vi "HFRR ADV v01.vi"() -> ()   [LabVIEW 2023] (continued)
5.386904015272106, 5.52926545136433, 5.687444824800141, 5.8368364552672976, 5.9967733772968375, 6.30610192979353, 6.478341691979186, 6.643551259789921, 6.808760827600658, 6.965182652442734, 7.137422414628394, 7.29032914228301, 7.492447230562097, 7.636566215248059, 7.747291776653125, 7.900198504307739, 8.067165620712203, 8.197224216648312, 8.429220631020835, 8.585642455862914, 8.749094475079918, 8.949455014765274, 9.075998513513923, 9.239450532730922, 9.40817519772912, 9.559324376790004, 9.675322583976262, 9.866895380692966, 9.9758633935043, 10.13580031553384, 10.293979688969653, 10.429310930686956, 10.59276294990396, 10.649004504903356, 10.823001815682744, 10.90209150240065, 11.049725584274075, 11.228995540834658, 11.366084331145693, 11.508445767237916, 11.642019460361494, 11.768562959110136, 11.905651749421176, 12.065588671450715, 12.241343530823832, 12.371402126759948, 12.585823055195151, 12.606913638319927, 12.867030830192144, 13.185147125657501, 13.396052956905242, 13.603443690965518, 13.83192500815058, 14.789788991734092, 17.011330414210352, 16.030618298908333, 15.981406938283856, 16.07455701375161, 15.802136981723274, 15.800379433129542, 16.00425507000236, 16.248554324531, 16.299523233749206, 16.77757645124409, 17.11151068405303, 16.812727423118723, 17.187085273583474, 16.94630111624229, 17.89713490545088, 18.072889764823994, 17.842650899045214, 17.6563507481097, 17.695016817171783, 17.872529225138642, 17.911195294200724, 17.890104711075956, 18.043011438730566, 17.958649106231476, 18.048284084511764, 18.072889764823994, 18.004345369668485, 18.148464354354438, 18.1801002290416, 18.17131248607295, 18.25040217279085, 18.257432367165777, 18.31367392216517, 18.35058244263353, 18.403308900445467, 18.41561174060159, 18.392763608883076, 18.459550455444862, 18.4841561357571, 18.507004267475608, 18.51930710763173, 18.57203356544366, 18.58960905138097, 18.619487377474403, 18.642335509192907, 18.64936570356783, 18.60718453731829, 18.605426988724552, 18.59839679434963, 18.57730621122485, 18.59488169716217, 18.56500337106873, 18.55797317669381, 18.57027601684993, 18.56676091966247, 18.531609947787846, 18.538640142162766, 18.528094850600382, 18.521064656225455, 18.52985239919411, 18.5122769132568, 18.482398587163367, 18.605426988724552, 18.614214731693213, 18.56148827388127, 18.56500337106873, 18.57203356544366, 18.549185433725157, 18.540397690756503, 18.52985239919411, 18.52985239919411, 18.5122769132568, 18.51403446185053, 18.515792010444265, 18.482398587163367, 18.494701427319487, 18.475368392788447, 18.464823101226052, 18.443732518101285, 18.459550455444862, 18.44900516388247, 18.427914580757704, 18.45076271247621, 18.436702323726358, 18.42439948357024, 18.433187226538898, 18.427914580757704, 18.408581546226657, 18.41385419200785, 18.389248511695616, 18.398036254664273, 18.38573341450815, 18.38221831732069, 18.38221831732069, 18.35058244263353, 18.368157928570838, 18.348824894039797, 18.34706734544607, 18.340037151071144, 18.331249408102487, 18.327734310915027, 18.31543147075891, 18.31543147075891, 18.301371082009055, 18.287310693259204, 18.297855984821588, 18.280280498884274, 18.275007853103087, 18.269735207321887, 18.25567481857205, 18.252159721384576, 18.232826686853535, 18.239856881228466, 18.215251200916224, 18.217008749509954, 18.209978555135034, 18.19064552060399, 18.195918166385184, 18.183615326229067, 18.169554937479216, 18.17307003466668, 18.153737000135635, 18.151979451541898, 18.137919062792054, 18.125616222635934, 18.12737377122967, 18.115070931073546, 18.115070931073546, 18.10276809091743, 18.099252993729966, 18.095737896542506, 18.09046525076131, 18.081677507792655, 18.067617119042804, 18.062344473261614, 18.055314278886687, 18.044768987324296, 18.03598124435564, 18.032466147168176, 18.023678404199522, 18.025435952793252, 18.021920855605796, 18.00961801544967, 17.99907272388729, 17.997315175293558, 17.99204252951236, 17.98501233513744, 17.97095194638759, 17.963921752012663, 17.958649106231476, 17.953376460450276, 17.946346266075352, 17.934043425919235, 17.93580097451296, 17.97095194638759, 17.953376460450276, 17.955134009044006, 17.94283116888789, 17.93931607170043, 17.927013231544308, 17.921740585763114, 17.891862259669683, 17.895377356857146, 17.89889245404461, 17.893619808263416, 17.881316968107296, 17.88307451670103, 17.879559419513566, 17.865499030763715, 17.833863156076553, 17.837378253264013, 17.80925747576432, 17.796954635608202, 17.796954635608202, 17.78465179545208, 17.77234895529596, 17.767076309514763, 17.777621601077154, 17.774106503889694, 17.742470629202533, 17.768833858108493, 17.719622497484025, 17.724895143265222, 17.724895143265222, 17.7178649488903, 17.728410240452682, 17.707319657327908, 17.70028946295298, 17.716107400296565, 17.703804560140444, 17.677441331234476, 17.65107810232851, 17.66865358826582, 17.5772610613918, 17.53859499232971, 17.52277705498613, 17.52453460357986, 17.515746860611202, 17.51047421483001, 17.50871666623628, 17.49992892326762, 17.491141180298964, 17.480595888736577, 17.477080791549124, 17.466535499986733, 17.464777951393007, 17.45423265983061, 17.44720246545569, 17.43314207670584, 17.43489962529957, 17.43138452811211, 17.419081687955984, 17.4085363963936, 17.403263750612407, 17.403263750612407, 17.390960910456286, 17.38744581326883, 17.382173167487633, 17.368112778737785, 17.368112778737785, 17.35405238998793, 17.347022195613008, 17.34174954983182, 17.339992001238087, 17.329446709675697, 17.325931612488237, 17.31714386951958, 17.308356126550922, 17.304841029363462, 17.303083480769722, 17.29429573780107, 17.278477800457495, 17.2732051546763, 17.26969005748884, 17.26265986311391, 17.257387217332717, 17.252114571551527, 17.245084377176603, 17.239811731395402, 17.23805418280167, 17.223993794051825, 17.223993794051825, 17.22047869686436, 17.213448502489445, 17.209933405301975, 17.20290321092705, 17.192357919364667, 17.188842822177204, 17.178297530614817, 17.17478243342735, 17.15720694749004, 17.146661655927648, 17.14490410733392, 17.136116364365265, 17.12908616999034, 17.122055975615414, 17.113268232646764, 17.178297530614817, 17.162479593271232, 17.115025781240494, 17.08338990655333, 17.081632357959595, 17.081632357959595, 17.067571969209745, 17.067571969209745, 17.06054177483482, 17.05702667764736, 17.051754031866164, 17.042966288897507, 17.035936094522594, 17.02363325436647, 17.01484551139781, 17.00957286561662, 16.995512476866768, 16.991997379679308, 16.990239831085574, 16.98496718530438, 16.979694539523184, 16.977936990929454, 16.96387660217961, 16.95508885921095, 16.951573762023486, 16.94278601905482, 16.933998276086164, 16.933998276086164, 16.92169543593005, 16.91642279014886, 16.9129076929614, 16.91642279014886, 16.904119949992744, 16.897089755617817, 16.895332207024087, 16.88654446405543, 16.87775672108677, 16.883029366867966, 16.867211429524385, 16.858423686555728, 16.85490858936826, 16.846120846399604, 16.832060457649764, 16.83030290905603, 16.823272714681107, 16.81624252030618, 16.810969874524982, 16.802182131556325, 16.8004245829626, 16.789879291400208, 16.789879291400208, 16.781091548431554, 16.768788708275437, 16.770546256869167, 16.767031159681704, 16.756485868119317, 16.754728319525583, 16.745940576556933, 16.738910382182006, 16.733637736400812, 16.724849993432162, 16.716062250463505, 16.702001861713647, 16.69672921593246, 16.698486764526187, 16.684426375776336, 16.682668827182606, 16.677396181401413, 16.666850889839022, 16.661578244057836, 16.659820695464106, 16.64927540390171, 16.640487660933058, 16.633457466558134, 16.628184820776944, 16.622912174995744, 16.622912174995744, 16.615881980620824, 16.60533668905843, 16.600064043277243, 16.59830649468351, 16.5807310087462, 16.577215911558728, 16.573700814371275]
  in  "ENTER THE NEW PASSWORD":string caption="Enter The New Password"
  in  "ENTER CURRENT PASSWORD":string caption="Enter Current Password"
  out "Port 3 Error":errorcluster
  in  "Lubrication System COM Port :":refnum<visa-resource-name>="COM9" caption="Ambient Temperature COM Port:"
  in  "LvdtOff":dbl=2.875 caption="LVDT Position Offset :" min=2.1 max=2.9 format="%.4f"
  out "Port 2 Error":errorcluster={"status"=TRUE, "code"=-1073807343, "source"="Property Node (arg 1) in VISA Configure Serial Port (Instr).vi->Winducom 2010--std ed hfrr-wo1768-V18.vi"}
  out "Port 1 Error":errorcluster={"status"=TRUE, "code"=-1073807343, "source"="Property Node (arg 1) in VISA Configure Serial Port (Instr).vi->Winducom 2010--std ed hfrr-wo1768-V18.vi"}
  in  "Stroke PID Gains":T9={"Proportional Gain (Kc)"=200.0, "Integral Time (Ti, min)"=0.02, "Derivative Time (Td, min)"=0.0}
  in  "CH-HUMIDITY DRY":u16=3 caption="Ch-Humidity Wet:" max=7 step=1
  in  "CH-HUMIDITY WET":u16=4 caption="Ch-Humidity Dry:" max=7 step=1
  in  "CH-HEATER":u16=2 caption="Ch-Heater:" max=7 step=1
  in  "CH-POWER -":u16=1 caption="Ch-Power -:" max=7 step=1
  in  "CH-POWER +":u16 caption="Ch-Power +:" max=7 step=1
  out "String 4":string
  in  "Com Port 3":refnum<visa-resource-name>="COM4" caption="Port 3"
  in  "Prog Due":bool
  in  "Prog Uno":bool
  in  "Com Port 2":refnum<visa-resource-name>="COM7" caption="Port 2:"
  in  "Com Port 1":refnum<visa-resource-name>="COM5" caption="Port 1:"
  in  "message":string="*Entered password is wrong"
  in  "SPEED OUT:":dbl=1.0 caption="Speed Out:" min=0.0001 max=5.0 step=0.0001 format="%.4f"
  in  "Temperature before test 3":dbl caption="Temp Before Test" format="%#_5g"
  in  "Humidity before test 3":dbl caption="Humidity Before Test" format="%#_5g"
  out "Temperature after test 5":dbl caption="Temp Before Test" format="%#_5g"
  out "Temperature after test 4":dbl caption="Temp After Test" format="%#_5g"
  out "Humidity after test 4":dbl caption="Humidity After Test ( % Rh )" format="%#_5g"
  out "Humidity before test 4":dbl caption="Humidity Before Test ( % Rh )" format="%#_5g"
  in  "Tab Control 9":enum32{"Page 1", "Page 2"}(tab)
  out "Ref B Scar Value :":string caption="Reference Fluid Information"
  out "Ref B Test Date :":string caption="Reference Fluid Information"
  out "Ref A Scar Value :":string caption="Reference Fluid Information"
  out "Ref A Test Date :":string caption="Reference Fluid Information"
  out "XY Graph 16":cluster{dbl[], dbl[]}[](graph)
  out "TITTLE 4":string caption="Reference Fluid Information"
  out "Sample ID  7":string caption="Fuel Name :"
  out "Sample ID  6":string caption="Fuel Type :"
  out "Mean Wear ( microns) :":dbl format="%#.6f"
  out "Wear Scar Y ( microns ) :":dbl format="%#.6f"
  out "Length ( microns ) 2":dbl caption="Wear Scar X ( microns ) :" format="%#.6f"
  out "s.NO 2":string caption="Instrument  S.NO :"
  out "Test Date 2":string caption="Tested date :"
  out "Tested by 2":string caption="Tested by :"
  out "Sample ID  2":string caption="Sample ID :"
  out "TITTLE 2":string caption="File Name :"
  in  "EDIT 3":bool
  in  "Upload Rate (s)":dbl=1.0 min=0.5 max=5.0 step=0.5 format="%.1g"
  in  "Secret Key":string="22gKHnAGFaJhuNtaR9srYhcD6RQR8M7Zp2xk4ssPTuwGqWUBv7WxW7cXAFkFFbns"
  in  "Serial No":string="HFRR2391"
  in  "Model No":string="MD987654325"
  in  "Data File Name":string="JSON_Single_Point.JSON"
  in  "Path":path=path "C:/LAB-IQ-NXT"
  in  "Upld AR 2":bool
  in  "Sen.Upload Rate (s)":dbl=5.0 min=0.5 max=5.0 step=0.5 format="%.1g"
  in  "Run test 3":bool
  in  "Sensor File Name":string="JSON_Health.JSON"
  in  "Upld AR":bool
  in  "Total No. of Tests":dbl
  in  "Tab Control 6":enum32{"Data", "Sensor"}(tab)=enum."Sensor"
  out "Respose From Server":string
  out "standard output":string
  out "SinglePoint":string
  in  "JSON Check String":string="\"Stored\": true"
  in  "JSONH Check String":string="\"Stored\": true"
  out "standard output 2":string
  in  "Sensor Information":string[][](array[string])=[["Sensor Name", "Sensor Model Number", "Sensor Run time Hours", "Sensor State"], ["Normal Load Sensor", "MPF-AC20-X3U791", "", ""], ["Frictional Force Sensor", "MPF-AC20-X3U792", "", ""], ["Temperature Sensor", "MPF-AC20-X3U793", "", ""], ["Speed Sensor", "MPF-AC20-X3U794", "", ""], ["LVDT Sensor", "MPF-AC20-X3U795", "", ""], ["Vibration Sensor ", "MPF-AC20-X3U796", "", ""]]
  out "Respose From Server 2":string
  out "FF buffer":dbl[](graph)
  out "%  o/p":dbl
  out "sample4":dbl format="%_4f"
  out "freq 4":dbl format="%_4f"
  out "conststatus":dbl=10.0 min=0.0 max=200.0 step=1.0
  out "CP4":dbl=nan min=0.0 max=200.0 step=0.1 format="%.3f"
  out "CP3":dbl=nan min=0.0 max=200.0 step=0.1 format="%.3f"
  out "Boolean  4":bool=TRUE caption="Power Status"
  in  "Boolean BC T & BG 2":cluster{u32, u32}[](array[cluster])=[{3158064, 16250871}, {11918296, 8965631}]
  in  "GBG   2":u32(colorbox)=16250871 caption="Graph Background"
  in  "GFG  2":u32(colorbox)=8964095 caption="Graph Foreground"
  in  "GBG":u32(colorbox)=16250871 caption="Graph Background"
  in  "GFG":u32(colorbox)=8964095 caption="Graph Foreground"
  in  "Boolean BC T & BG":cluster{u32, u32}[](array[cluster])=[{3158064, 16250871}, {11918296, 8965631}]
  in  "SC  Text":u32(colorbox) caption="String Control Text"
  in  "SC BG 3":u32(colorbox)=16777215 caption="String Control BG"
  in  "NI BG 2":u32(colorbox)=13553358 caption="Numeric Indicator BG"
  in  "NI Text  2":u32(colorbox)=7105644 caption="Numeric Indicator Text"
  in  "NC Text":u32(colorbox)=3381759 caption="Numeric Control Text"
  in  "NC BG":u32(colorbox)=16777215 caption="Numeric Control BG"
  out "ABS DP":dbl[](graph)
  in  "Com flag":u32
  out "Gain path":string="C:\\Winducom 2010\\STD ED HFRR\\wo1768"
  out "String 45":string="S.NO"
  out "String 44":string
  out "error out 4":errorcluster
  out "concatenated string 2":string
  out "String 42":string
  out "error out 3":errorcluster
  out "STR":string
  out "gain":string
  out "export":string
  out "before substring":string
  out "output":string
  out "test by":string
  out "export 2":string
  out "export":string
  out "REMARKS 2":string="@WINDUCOM : RECIPROCATORY TEST RIG    DEFINITON FILE       \r  Sample ID :- , Load :-  2.00 N , Remarks :- , Date :- 05/11/2016, 06:04\r"
  out "data":string
  out "Boolean 3":bool
  out "String 41":string=":-@(WINDUCOM : RECIPROCATORY TEST RIG    DEFINITON FILE )      "
  out "concatenated string":string
  out "path":path
  out "String 40":string
  out "Boolean 2":bool=TRUE
  in  "Set Rh 2":dbl=50.0 caption="HUMIDITY" min=35.0 max=85.0 step=1.0
  out "String 39":string="WS1.4="
  out "String 38":string="HCF="
  out "String 37":string="MWSD="
  out "String 36":string="AVP ="
  out "String 35":string="Temp after test="
  out "String 34":string="Temp before test="
  out "String 33":string="Tested by"
  out "String 32":string="Sample ID "
  out "String 31":string="Tested date"
  out "String 30":string="Sample Design"
  out "path string":string
  out "String 29":string
  out "St. Line eqn : 2":string
  out "Numeric 10":i32
  out "Numeric 16":i32
  out "S 106":string="Off"
  out "S 105":string="On"
  out "S 104":string="Heater Off"
  out "S 103":string="Heater On"
  out "S 102":string="Ch-Humidity Dry:"
  out "S 101":string="Ch-Humidity Wet:"
  out "S 100":string="Ch-Heater:"
  out "S 99":string="Ch-Power -:"
  out "S 98":string="Ch-Power +:"
  out "S 97":string="Port 2"
  out "S 96":string="Port 1"
  out "S 95":string="Stroke Gain :"
  out "S 94":string="Displacement :"
  out "S 93":string="Stop"
  out "S 92":string="Run"
  in  "LAnguage":enum32{"Page 1", "Page 2"}(tab)
  out "S 91":string="Threshold"
  out "S 90":string="File path"
  out "S 89":string="Newtons ( N )"
  out "S 88":string="Change Calibrate Password"
  out "S 87":string="Enter The New Password"
  out "S 86":string="Enter Current Password"
  out "S 85":string="Password"
  out "S 84":string="Save Gain Constants"
  out "S 83":string="Air Temperature ( deg C )"
  out "S 82":string="TIME ( mins )"
  out "S 81":string="Relative Humidity ( Rh )"
  out "S 80":string="Sample TEMPERATURE ( Deg C)"
  out "S 79":string="Stroke"
  out "S 78":string="Air Temperature"
  out "S 77":string="mm"
  out "S 76":string="Stroke"
  out "S 75":string="WINDUCOM 2010 \\XXXX\\VX.XX\\MONTH YEAR"
  out "S 74":string="Frictional Force ( N )"
  out "S 73":string="Calibrate Parameter"
  out "S 72":string="Save Gain Constant"
  out "S 71":string="Edit Gain Constant"
  out "S 70":string="Humidity :"
  out "S 69":string="Air Temperature :"
  out "S 68":string="Speed Out:"
  out "S 67":string="Temperature :"
  out "S 66":string="Frictional Force :"
  out "S 65":string="ABOUT"
  out "S 64":string="Frictional  Force ( N )"
  out "S 63":string="Temperature ( Deg C)"
  out "S 62":string="Time ( mins )"
  out "S 60":string="Reset Graph"
  out "S 59":string="COF4"
  out "S 58":string="COF3"
  out "S 57":string="COF2"
  out "S 56":string="COF1"
  out "S 55":string="Frictional Force ( N )"
  out "S 54":string="Temperature"
  out "S 53":string="Coefficient Of Friction"
  out "S 52":string="Refresh"
  out "S 51":string="File 4"
  out "S 50":string="File 3"
  out "S 49":string="File 2"
  out "S 48":string="File 1"
  out "S 47":string="COMPARE FILES"
  out "S 46":string="SAVE RESULT"
  out "S 45":string="WS1.4"
  out "S 44":string="HCF"
  out "S 43":string="MWSD"
  out "S 42":string="AVP "
  out "S 41":string
  out "S 40":string
  out "S 39":string="Humidity after test="
  out "S 38":string="Humidity before test="
  out "S 37":string
  out "S 36":string="Rh Before"
  out "S 35":string="ISO : WS1.4"
  out "S 34":string="FRICTIONAL FORCE ( N )"
  out "S 33":string="Reset Graph"
  out "S 32":string="Data points"
  out "S 31":string="COEFFICIENT OF FRICTION"
  out "S 30":string="RUN"
  out "S 29":string="Test Status"
  out "S 28":string="Power"
  out "S 27":string="Engage"
  out "S 26":string="Present ( Sec )"
  out "S 25":string="Count down ( sec )"
  out "S 24":string="Sec"
  out "S 23":string="Save Dwell"
  out "S 22":string="Elapsed Time"
  out "S 21":string="min"
  out "S 20":string="Test duration"
  out "S 19":string="TIMER"
  out "S 18":string="OFF"
  out "S 17":string="Rh"
  out "S 16":string="HUMIDITY"
  out "S 15":string="Heater On"
  out "S 14":string="TEMPERATURE ( Deg C)"
  out "S 13":string="N"
  out "S 12":string="NORMAL LOAD"
  out "S 11":string="Hz"
  out "S 10":string="FREQUENCY"
  out "S 9":string="STOP"
  out "S 8":string="STAND BY"
  out "S 7":string="Remarks :"
  out "S 6":string="Sample ID :"
  out "S 5":string="File Name :"
  out "S 4":string="Acquire"
  out "S 3":string="EXIT"
  out "S 2":string="Winducom 2010"
  out "S":string="ENGLISH TITLES"
  out "Error Due":errorcluster={"status"=TRUE, "code"=-1073807343, "source"="Property Node (arg 1) in VISA Configure Serial Port (Instr).vi->Winducom 2010--std ed hfrr-wo1768-V18.vi"}
  out "Error Uno":errorcluster={"status"=TRUE, "code"=-1073807343, "source"="Property Node (arg 1) in VISA Configure Serial Port (Instr).vi->Winducom 2010--std ed hfrr-wo1768-V18.vi"}
  out "as":string
  out "bs":string="Rh After"
  out "as":string=" after test"
  out "bs":string="Temp"
  out "as":string=" before test"
  out "bs":string="Temp"
  out "as":string=" after test"
  out "bs":string
  out "bs":string="Humidity"
  out "as":string=" before test"
  out "bs":string="Humidity"
  out "S 61":string="Frictional Force ( N )"
  in  "Lan flag":dbl=22.0
  in  "Table":string[][](table)=[["ENGLISH TITLES", "RUSSIAN"], ["Winducom 2010", "Winducom  2010"], ["Exit", "Выход"], ["Acquire", "ИСПЫТАНИЕ     "], ["File Name :", "Имя файла :"], ["Sample ID :", "Имя образца :"], ["Remarks :", "Примечания :"], ["Standby", "ОЖИДАНИЕ"], ["Stop", "СТОП"], ["Frequency", "ЧАСТОТА"], ["Hz", "Гц"], ["Normal Load", "НАГРУЗКА"], ["N", "Н"], ["Temperature ( Deg C)", "ТЕМПЕРАТУРА (Град С)"], ["Heater On", "НАГРЕВ ВКЛ"], ["Humidity", "ВЛАЖНОСТЬ"], ["Rh", "%"], ["OFF", "ВЫКЛ"], ["Timer", "ВРЕМЯ"], ["Test duration", "ВРЕМЯ ТЕСТА"], ["min", "мин"], ["Elapsed Time", "依商判"], ["Save Dwell", "ИНТЕРВАЛ"], ["Sec", "Сек"], ["Count down ( Sec )", "До запуска (сек)"], ["Present ( Sec )", "Таймер (сек)"], ["Run", "Применить"], ["Power", "ПИТАНИЕ"], ["Test Status", "СТАТУС"], ["Manual Over Ride", "ПУСК"], ["Coefficient Of Friction", "КОЭФФИЦИЕНТ ТРЕНИЯ"], ["Data points", "Точки"], ["Reset Graph", "Сбросить график"], ["Frictional Force ( N )", "СИЛА ТРЕНИЯ (Н)"], ["ISO : WS1.4", "ISO : WS1.4"], ["Rh Before", "Влажность до"], ["Rh After", "Влажность, после"], ["Humidity, before test", "Влажность, до теста"], ["Humidity, after test", "Влажность, после теста"], ["Temp, before test", "Температура, до теста"], ["Temp, after test", "Температура, после теста"], ["AVP ", "СДП"], ["MWSD", "MWSD"], ["HCF", "ФКВ"], ["WS1.4", "WS1.4"], ["Save Result", "Сохранить результат"], ["COMPARE FILES", ""], ["File 1", "ФАЙЛ 1"], ["File 2", "ФАЙЛ 2"], ["File 3", "ФАЙЛ 3"], ["File 4", "ФАЙЛ 4"], ["Refresh", "ОБНОВИТЬ"], ["Coefficient Of Friction", "КОЭФФИЦИЕНТ ТРЕНИЯ"], ["Temperature", "ТЕМПЕРАТУРА"], ["Frictional Force ( N )", "СИЛА ТРЕНИЯ (Н)"], ["COF1", "КОФ1"], ["COF2", "КОФ2"], ["COF3", "КОФ3"], ["COF4", "КОФ4"], ["Reset Graph", "Сбросить график"], ["Time ( mins )", "Время (мин)"], ["Temperature ( Deg C)", "ТЕМПЕРАТУРА (Град С)"], ["Frictional  Force ( N )", "СИЛА ТРЕНИЯ (Н)"], ["ABOUT", ""], ["Frictional Force :", "КОЭФ.ТРЕНИЯ:"], ["Temperature :", "ТЕМПЕРАТУРА"], ["Speed Out:", "СКОРОСТЬ"], ["Air Temperature :", "ТЕМПЕРАТУРА ВОЗДУХА"], ["Humidity :", "ВЛАЖНОСТЬ"], ["Edit Gain Constant", "КОРРЕКТИРОВКА КОНСТАНТ"], ["Save Gain Constant", "СОХРАНИТЬ КОНСТАНТЫ"], ["Calibrate Parameter", "ПАРАМЕТРЫ КАЛИБРОВКИ"], ["Frictional Force ( N )", "СИЛА ТРЕНИЯ (Н)"], ["WINDUCOM 2010 \\XXXX\\VX.XX\\MONTH YEAR", "WINDUCOM 2010 \\XXXX\\VX.XX\\MONTH YEAR"], ["Stroke", "ДЛИННА ХОДА"], ["mm", "мм"], ["Air Temperature", "ВОЗДУХА ТЕМП"], ["Stroke", "ДЛИННА ХОДА "], ["Time ( mins )", "ВРЕМЯ ( мин )"], ["Sample Temperature( Deg C)", "Образец ТЕМПЕРАТУРА (Град С)"], ["Relative Humidity ( Rh )", "Относительный Влажность ( % )"], ["Air Temperature ( deg C )", "ТЕМПЕРАТУРА ВОЗДУХА (Град С)"], ["Save Gain Constants", "СОХРАНИТЬ КОНСТАНТЫ"], ["Password", "ПАРОЛЬ ДОСТУПА"], ["Enter Current Password", "ВВЕДИТЕ ТЕКУЩИЙ ПАРОЛЬ"], ["Enter The New Password", "ВВЕДИТЕ НОВЫЙ ПАРОЛЬ"], ["Change Calibrate Password", "Сбросить пароль калибровки"], ["Newtons ( N )", "Ньютон ( Н )"], ["File path", "Путь к файлу"], ["Threshold", "порог"], ["Run", "ПУСК"], ["Stop", "СТОП"], ["Displacement :", "смещение:"], ["Stroke Gain :", "ДЛИННА ХОДА:"], ["Port 1", "порт 1"], ["Port 2", "порт 2"], ["Ch-Power +:", "CH-ПИТАНИЕ +:"], ["Ch-Power -:", "CH-ПИТАНИЕ -:"], ["Ch-Heater:", "НАГРЕВ:"], ["Ch-Humidity Wet:", "CH-Увлажнение:"], ["Ch-Humidity Dry:", "CH-Осушение:"], ["Heater On", "НАГРЕВ ВКЛ"], ["Heater Off", "НАГРЕВ ВЫКЛ"], ["On", "ВКЛ"], ["Off", "ВЫКЛ"], ["TEXT REPORT", "ПРОТОКОЛ ИСПЫТАНИЯ"], ["Open Data File", "ОТКРЫТЬ ФАЙЛ ДАННЫХ"], ["Refresh", "ОБНОВЛЕНО"], ["Tittle", "заглавие"], ["Sample Design", "Образец"], ["Tested date", "Дата"], ["Sample ID ", "Имя образца"], ["Tested by", "Испытано"], ["System Configured Printers ", "Сконфигурированные принтеры"], ["Selected Printer", "Выбранный принтер"], ["Select Printer 3", "Выбрать  Печать"], ["Print", "Печать"], [":-@(WINDUCOM : RECIPROCATORY TEST RIG    DEFINITON FILE )      ", "(Анализатор HFRR с возвратно-поступательным механизмом для определения смазывающей способности дизельных топлив )"], ["Tested by:", "Оператор:"], ["          TIME;      COF;       STROKE  (mm);     AIR TEMP ( Deg C);  TEMP ( Deg C);  HUMIDITY ( Rh );", "КОЭФФИЦИЕНТ ТРЕНИЯ;   Инсульт; ТЕМПЕРАТУРА ВОЗДУХА; ВЛАЖНОСТЬ;"], ["Export", "Экспорт"], ["Temperature Intercept :", "ТЕМП перехват:"], ["Air Temperature Intercept:", "ТЕМП  ВОЗДУХА перехват:"], ["Select File Type ", "Выберете формат файла"], ["S.NO", "S.NO"], ["Trip", ""]]
  out "Fric Val":dbl[](array[numeric])
  out "FF cal val":dbl[](array[numeric])=[-0.013084344151737926, -0.01288606647100253, -0.011498122705853597, -0.012092955748060075, -0.011101567344382515, -0.011696400386589284, -0.010705011982911433, -0.010110178940704664, -0.011498122705853597, -0.01090328966364712, -0.009911901259969269, -0.009911901259969269, -0.009515345898498478, -0.008523957494820628, -0.008127402133349837, -0.008127402133349837, -0.009118790537027396, -0.008325679814085232, -0.008325679814085232, -0.008523957494820628, -0.008325679814085232, -0.008127402133349837, -0.008523957494820628, -0.00792912445261415, -0.008325679814085232, -0.008325679814085232, -0.007730846771878755, 0.0015882042226915277, -0.0027739047534900835, -0.0059463476452584485, -0.007136013729671986, -0.006739458368200904, -0.008325679814085232, -0.008523957494820628, -0.007334291410407381, -0.007730846771878755, -0.007334291410407381, -0.007136013729671986, -0.00792912445261415, -0.007334291410407381, -0.006937736048936299, -0.006342903006729822, -0.006342903006729822, -0.006342903006729822, -0.006144625325994427, -0.006144625325994427, -0.0055497922837873664, -0.004954959241580889, -0.005351514603051971, -0.004954959241580889, -0.004954959241580889, -0.004161848518639016, -0.003170460114961457, -0.0023773493920190014, -0.0023773493920190014, -0.0019807940305479194, -0.0019807940305479194, -0.0011876833076060467, -0.0009894056268700685, -0.0009894056268700685, -0.0009894056268700685, -0.0007911279461346732, -0.00019629490392819582, 0.00020026045754288624, 0.0007950934997493636, 0.001389926541955841, 0.0021830372648982965, 0.0033727033493112513, 0.004165814072253707, 0.0037692587107826248, 0.0037692587107826248, 0.004165814072253707, 0.0049589247951955795, 0.005752035518137744, 0.006346868560344221, 0.007338256964022072, 0.007734812325493154, 0.008726200729171005, 0.010510699855790728, 0.00991586681358396, 0.011105532897997497, 0.011502088259468288, 0.012096921301675348, 0.012493476663146139, 0.01289003202461722, 0.01289003202461722, 0.014277975789765862, 0.015269364193443713, 0.016260752597121272, 0.01745041868153452, 0.018243529404476683, 0.019036640127418555, 0.018640084765947473, 0.01982975085036101, 0.020028028531096406, 0.021415972296245048, 0.021415972296245048, 0.0224073606999229, 0.023002193742129376, 0.02379530446507154, 0.024984970549484786, 0.025579803591691264, 0.024984970549484786, 0.02538152591095587, 0.025976358953162346, 0.026571191995369114, 0.027166025037575592, 0.027959135760518047, 0.027959135760518047, 0.02875224648345963, 0.029545357206402084, 0.03033846792934425, 0.03033846792934425, 0.030933300971550726, 0.0313298563330221, 0.03212296705596397, 0.03271780009817045, 0.03291607777890643, 0.03470057690552586, 0.034502299224790464, 0.03529540994773234, 0.03668335371288127, 0.036485076032145874, 0.0380712974780302, 0.03727818675508775, 0.03787301979729481, 0.04659723774965803, 0.0406489073275918, 0.04025235196612072, 0.04005407428538532, 0.04104546268906317, 0.041442018050534254, 0.04699379311112911, 0.05155417976804641, 0.05314040121393045, 0.05333867889466584, 0.05433006729834369, 0.05452834497907909, 0.057700787870848036, 0.055718011063492626, 0.047786903834071276, 0.04461446094230262, 0.043821350219360164, 0.043821350219360164, 0.04362307253862477, 0.04421790558083154, 0.04461446094230262, 0.0452092939845091, 0.0450110163037737, 0.0452092939845091, 0.045804127026715866, 0.04600240470745155, 0.04639896006892234, 0.04719207079186451, 0.047390348472600194, 0.04798518151480696, 0.04858001455701315, 0.04937312527995531, 0.05016623600289748, 0.05135590208731072, 0.05135590208731072, 0.05135590208731072, 0.05135590208731072, 0.05155417976804641, 0.05254556817172426, 0.051752457448781805, 0.05155417976804641, 0.05214901281025318, 0.0519507351295172, 0.051752457448781805, 0.05333867889466584, 0.052347290490988574, 0.05254556817172426, 0.05294212353319505, 0.05393351193687261, 0.05393351193687261, 0.053735234256137215, 0.05393351193687261, 0.0541317896176083, 0.054726622659814775, 0.055321455702021544, 0.05551973338275694, 0.05591628874422802, 0.05710595482864156, 0.057304232509376954, 0.05849389859378991, 0.05829562091305422, 0.057700787870848036, 0.05750251019011235, 0.058097343232318535, 0.057304232509376954, 0.057700787870848036, 0.05789906555158343, 0.058097343232318535, 0.058692176274525595, 0.058692176274525595, 0.05928700931673207, 0.05948528699746776, 0.05948528699746776, 0.06087323076261669, 0.06047667540114561, 0.06047667540114561, 0.06087323076261669, 0.06087323076261669, 0.06126978612408748, 0.06126978612408748, 0.06186461916629425, 0.06245945220850073, 0.06206289684702965, 0.06186461916629425, 0.06186461916629425, 0.062261174527765334, 0.06206289684702965, 0.06206289684702965, 0.0632525629314429, 0.06285600756997181, 0.06364911829291427, 0.0630542852507072, 0.06285600756997181, 0.06245945220850073, 0.06265772988923642, 0.06285600756997181, 0.06364911829291427, 0.06384739597364966, 0.06384739597364966, 0.06384739597364966, 0.06384739597364966, 0.06464050669659183, 0.06503706205806291, 0.0652353397387986, 0.06483878437732722, 0.06543361741953399, 0.0652353397387986, 0.0652353397387986, 0.06503706205806291, 0.06563189510026968, 0.06602845046174047, 0.06682156118468263, 0.0676146719076245, 0.06880433799203804, 0.07851994434807912, 0.08149410955911209, 0.0721750585645418, 0.07138194784159993, 0.07019228175718698, 0.07019228175718698, 0.07078711479939345, 0.07019228175718698, 0.07138194784159993, 0.07197678088380641, 0.07257161392601288, 0.07237333624527749, 0.07237333624527749, 0.07356300232969074, 0.0743561130526329, 0.0743561130526329, 0.07415783537189721, 0.07415783537189721, 0.0743561130526329, 0.0745543907333683, 0.07554577913704615, 0.07415783537189721, 0.0745543907333683, 0.07554577913704615, 0.07574405681778183, 0.07594233449851723, 0.07633888985998831, 0.0767354452214591, 0.0765371675407237, 0.07633888985998831, 0.07693372290219479, 0.0765371675407237, 0.0765371675407237, 0.07614061217925233, 0.07614061217925233, 0.07614061217925233, 0.07614061217925233, 0.0765371675407237, 0.07713200058293018, 0.07693372290219479, 0.07693372290219479, 0.07733027826366587, 0.07713200058293018, 0.0765371675407237, 0.0765371675407237, 0.07614061217925233, 0.0765371675407237, 0.0765371675407237, 0.07574405681778183, 0.07554577913704615, 0.07554577913704615, 0.07475266841410427, 0.07574405681778183, 0.0745543907333683, 0.07376128001042642, 0.07356300232969074, 0.07376128001042642, 0.07336472464895534, 0.07395955769116182, 0.0743561130526329, 0.07475266841410427, 0.07495094609483967, 0.0745543907333683, 0.0743561130526329, 0.07356300232969074, 0.07257161392601288, 0.07257161392601288, 0.07376128001042642, 0.07296816928748397, 0.07276989160674857, 0.07276989160674857, 0.07276989160674857, 0.07237333624527749, 0.07257161392601288, 0.07237333624527749, 0.07197678088380641, 0.07177850320307101, 0.07158022552233533, 0.07158022552233533, 0.07177850320307101, 0.07177850320307101, 0.07237333624527749, 0.07257161392601288, 0.07276989160674857, 0.07356300232969074, 0.07356300232969074, 0.07316644696821965, 0.07376128001042642, 0.07376128001042642, 0.0743561130526329, 0.07495094609483967, 0.07554577913704615, 0.07713200058293018, 0.07752855594440126, 0.07812338898660803, 0.07871822202881451, 0.07812338898660803, 0.07832166666734372, 0.08010616579396344, 0.08684760693897126, 0.08248549796278964, 0.08149410955911209, 0.08149410955911209, 0.08169238723984748, 0.08228722028205396, 0.08724416230044234, 0.09398560344545102, 0.09339077040324396, 0.09497699184912858, 0.09596838025280614, 0.09775287937942587, 0.09834771242163234, 0.10033048922898775, 0.1017184329941364, 0.10290809907854964, 0.10469259820516966, 0.10310637675928533, 0.10310637675928533, 0.10330465444002072, 0.10409776516296318, 0.10766676341620263, 0.10786504109693802, 0.1062788196510537, 0.1104426509465002, 0.10766676341620263, 0.10905470718135127, 0.11064092862723589, 0.10905470718135127, 0.10072704459045913, 0.0991408231445748, 0.09973565618678128, 0.09953737850604588, 0.09993393386751667, 0.10013221154825236, 0.10013221154825236, 0.09973565618678128, 0.10033048922898775, 0.10033048922898775, 0.10132187763266531, 0.10132187763266531, 0.10132187763266531, 0.10132187763266531, 0.10211498835560777, 0.10211498835560777, 0.1037012098014921, 0.10270982139781425, 0.10310637675928533, 0.1037012098014921, 0.10429604284369857, 0.10409776516296318, 0.10389948748222749, 0.10469259820516966, 0.10489087588590505, 0.10528743124737643, 0.10568398660884751, 0.10588226428958261, 0.10568398660884751, 0.106080541970318, 0.10647709733178909, 0.10766676341620263, 0.1062788196510537, 0.10687365269326046, 0.10687365269326046, 0.10707193037399586, 0.10707193037399586, 0.10687365269326046, 0.10687365269326046, 0.10727020805473154, 0.10766676341620263, 0.1082615964584091, 0.10806331877767342, 0.10845987413914479, 0.10865815181988048, 0.10964954022355804, 0.11004609558502883, 0.11064092862723589, 0.11143403935017776, 0.11143403935017776, 0.11143403935017776, 0.11222715007312022, 0.11242542775385561, 0.11183059471164913, 0.11163231703091345, 0.1126237054345913, 0.11302026079606209, 0.11341681615753346, 0.11381337151900454, 0.11420992688047533, 0.11520131528415319, 0.11460648224194613, 0.1150030376034175, 0.11599442600709506, 0.11539959296488858, 0.11559787064562398, 0.11599442600709506, 0.11599442600709506, 0.11599442600709506, 0.11678753673003751, 0.11678753673003751, 0.11698581441077291, 0.11658925904930183, 0.11738236977224399, 0.11797720281445047, 0.11698581441077291, 0.11658925904930183, 0.11738236977224399, 0.11639098136856614, 0.11658925904930183, 0.1171840920915086, 0.11738236977224399, 0.11758064745297939, 0.11777892513371507, 0.1263048654053432, 0.12828764221269862, 0.11936514657959911, 0.11857203585665724, 0.1171840920915086, 0.1171840920915086, 0.11698581441077291, 0.11639098136856614, 0.11738236977224399, 0.11738236977224399, 0.11777892513371507, 0.11797720281445047, 0.11797720281445047, 0.11797720281445047, 0.11857203585665724, 0.11797720281445047, 0.11758064745297939, 0.11758064745297939, 0.1171840920915086, 0.11658925904930183, 0.11698581441077291, 0.1171840920915086, 0.11639098136856614, 0.1171840920915086, 0.11619270368783075, 0.11738236977224399, 0.11639098136856614, 0.11658925904930183, 0.11678753673003751, 0.11698581441077291, 0.11658925904930183, 0.11658925904930183, 0.11877031353739292, 0.11758064745297939, 0.11678753673003751, 0.11658925904930183, 0.11619270368783075, 0.11579614832635966, 0.11599442600709506, 0.11520131528415319, 0.11579614832635966, 0.11460648224194613, 0.11460648224194613, 0.11480475992268181, 0.11401164919973965, 0.11381337151900454, 0.11381337151900454, 0.11361509383826915, 0.11361509383826915, 0.11420992688047533, 0.11420992688047533, 0.11460648224194613, 0.11460648224194613, 0.11480475992268181, 0.11539959296488858, 0.11440820456121073, 0.11460648224194613, 0.1150030376034175, 0.11480475992268181, 0.11480475992268181, 0.1150030376034175, 0.11539959296488858, 0.11579614832635966, 0.11539959296488858, 0.11639098136856614, 0.11579614832635966, 0.11658925904930183, 0.11698581441077291, 0.11758064745297939, 0.11877031353739292, 0.11837375817592184, 0.11837375817592184, 0.11896859121812803, 0.11916686889886342, 0.11976170194107048, 0.12015825730254127, 0.12075309034474804, 0.12134792338695452, 0.12233931179063237, 0.12313242251357454, 0.12352897787504562, 0.12432208859798749, 0.12511519932092965, 0.1263048654053432, 0.1261065877246072, 0.12670142076681398, 0.12749453148975615, 0.12709797612828505, 0.12689969844754967, 0.12769280917049153, 0.12828764221269862, 0.12987386365858264, 0.12987386365858264, 0.13027041902005343, 0.13086525206226018, 0.13205491814667344, 0.1324514735081445, 0.13225319582740885, 0.13264975118887992, 0.1330463065503513, 0.13899463697241693, 0.13701186016506184, 0.1401843030568302, 0.14553780043668996, 0.1467274665211029, 0.14752057724404535, 0.14989990941287126, 0.15406374070831777, 0.15446029606978856, 0.1556499621542021, 0.1554516844734664, 0.15664135055787964, 0.15723618360008643, 0.15822757200376397, 0.15902068272670586, 0.15941723808817693, 0.1600120711303837, 0.15882240504597045, 0.15981379344964802, 0.15822757200376397, 0.15862412736523507, 0.1602103488111194, 0.1600120711303837, 0.15921896040744155, 0.16040862649185478, 0.1602103488111194, 0.15644307287714398, 0.15426201838905318, 0.1536671853468467, 0.1532706299853756, 0.15465857375052425, 0.15426201838905318, 0.15426201838905318, 0.15426201838905318, 0.15426201838905318, 0.15406374070831777, 0.15426201838905318, 0.15386546302758208, 0.153468907666111, 0.15247751926243344, 0.15247751926243344, 0.15128785317802018, 0.1508912978165491, 0.15029646477434264, 0.14970163173213585, 0.14910679868992938, 0.14930507637066479, 0.14771885492478076, 0.1445464120330121, 0.1465291888403675, 0.1495033540514002, 0.14811541028625183, 0.14712402188257429, 0.14712402188257429, 0.1469257442018383, 0.14593435579816072, 0.14712402188257429, 0.14613263347889643, 0.14494296739448287, 0.14573607811742534, 0.14573607811742534, 0.14553780043668996, 0.1467274665211029, 0.14533952275595396, 0.1447446897137475, 0.1447446897137475, 0.14494296739448287, 0.14494296739448287, 0.14533952275595396, 0.14533952275595396, 0.14553780043668996, 0.14553780043668996, 0.14573607811742534, 0.1465291888403675, 0.1467274665211029, 0.1467274665211029, 0.14593435579816072, 0.14533952275595396, 0.1465291888403675, 0.1467274665211029, 0.1469257442018383, 0.1469257442018383, 0.14633091115963182, 0.14613263347889643, 0.1467274665211029, 0.1465291888403675, 0.1467274665211029, 0.14752057724404535, 0.14771885492478076, 0.14771885492478076, 0.1485119656477229, 0.14989990941287126, 0.14989990941287126, 0.14970163173213585, 0.14989990941287126, 0.15128785317802018, 0.15168440853949128, 0.15247751926243344, 0.15267579694316913, 0.1536671853468467, 0.1536671853468467, 0.15406374070831777, 0.15505512911199504, 0.15505512911199504, 0.15465857375052425, 0.15505512911199504, 0.15525340679273103, 0.1554516844734664, 0.1558482398349375, 0.15624479519640858, 0.15683962823861536, 0.15703790591935074, 0.15683962823861536, 0.16080518185332587, 0.1602103488111194, 0.15009818709360695, 0.14831368796698724, 0.14831368796698724, 0.14811541028625183, 0.14831368796698724, 0.1487102433284583, 0.1487102433284583, 0.14910679868992938, 0.1495033540514002, 0.15029646477434264, 0.15009818709360695, 0.1495033540514002, 0.1495033540514002, 0.14890852100919372, 0.14910679868992938, 0.14910679868992938, 0.14910679868992938, 0.14890852100919372, 0.14890852100919372, 0.14890852100919372, 0.1487102433284583, 0.14831368796698724, 0.14930507637066479, 0.14890852100919372, 0.1485119656477229, 0.14910679868992938, 0.14890852100919372, 0.14831368796698724, 0.1485119656477229, 0.1485119656477229, 0.1485119656477229, 0.1506930201358137, 0.1487102433284583, 0.14831368796698724, 0.14811541028625183, 0.14732229956330967, 0.14791713260551614, 0.14732229956330967, 0.14752057724404535, 0.14910679868992938, 0.14831368796698724, 0.14831368796698724, 0.14791713260551614, 0.14752057724404535, 0.14732229956330967, 0.1469257442018383, 0.14732229956330967, 0.14732229956330967, 0.14732229956330967, 0.1469257442018383, 0.14613263347889643, 0.1469257442018383, 0.1467274665211029, 0.14633091115963182, 0.14633091115963182, 0.14633091115963182, 0.14633091115963182, 0.14553780043668996, 0.1447446897137475, 0.1447446897137475, 0.1443481343522764, 0.14395157899080563, 0.144149856671541, 0.14395157899080563, 0.14335674594859885, 0.14315846826786344, 0.14315846826786344, 0.14335674594859885, 0.14395157899080563, 0.14315846826786344, 0.14256363522565696, 0.14296019058712806, 0.14177052450271452, 0.14137396914124345, 0.14097741377977263, 0.14077913609903697, 0.14097741377977263, 0.14077913609903697, 0.14058085841830126, 0.13998602537609478, 0.13998602537609478, 0.1395894700146237, 0.13919291465315264, 0.13919291465315264, 0.13859808161094617, 0.1376066932072686, 0.13839980393021076, 0.13780497088800397, 0.1376066932072686, 0.13780497088800397, 0.1374084155265329, 0.1376066932072686, 0.13820152624947507, 0.13839980393021076, 0.13879635929168127, 0.13899463697241693, 0.13839980393021076, 0.13839980393021076, 0.13879635929168127, 0.14256363522565696, 0.1423653575449213, 0.1403825807375656, 0.1401843030568302, 0.13978774769535912, 0.13998602537609478, 0.14097741377977263, 0.1506930201358137, 0.15029646477434264, 0.15168440853949128, 0.1532706299853756, 0.15465857375052425, 0.15525340679273103, 0.1576327389615575, 0.1558482398349375, 0.14732229956330967, 0.14593435579816072, 0.144149856671541, 0.14296019058712806, 0.14296019058712806, 0.14335674594859885, 0.14395157899080563, 0.144149856671541, 0.1445464120330121, 0.1445464120330121, 0.14533952275595396, 0.14553780043668996, 0.14553780043668996, 0.14533952275595396, 0.14553780043668996, 0.14553780043668996, 0.14613263347889643, 0.14593435579816072, 0.14732229956330967, 0.1465291888403675, 0.1465291888403675, 0.1465291888403675, 0.1467274665211029, 0.14712402188257429, 0.14831368796698724, 0.14752057724404535, 0.14752057724404535, 0.14752057724404535, 0.14732229956330967, 0.14732229956330967, 0.14811541028625183, 0.14831368796698724, 0.1485119656477229, 0.14989990941287126, 0.15029646477434264, 0.15029646477434264, 0.15029646477434264, 0.15029646477434264, 0.14970163173213585, 0.15009818709360695, 0.14970163173213585, 0.1495033540514002, 0.15009818709360695, 0.14989990941287126, 0.14989990941287126, 0.1506930201358137, 0.1506930201358137, 0.15128785317802018, 0.1514861308587556, 0.15168440853949128, 0.15188268622022666, 0.15227924158169803, 0.15247751926243344, 0.15247751926243344, 0.1532706299853756, 0.15406374070831777, 0.15406374070831777, 0.15406374070831777, 0.15505512911199504, 0.1554516844734664, 0.15644307287714398, 0.15664135055787964, 0.15723618360008643, 0.15703790591935074, 0.1578310166422929, 0.15743446128082184, 0.15743446128082184, 0.1578310166422929, 0.15743446128082184, 0.1576327389615575, 0.1578310166422929, 0.1580292943230283, 0.15862412736523507, 0.15921896040744155, 0.1600120711303837, 0.16080518185332587, 0.16140001489553263, 0.1623914032992102, 0.1623914032992102, 0.16298623634141668, 0.16318451402215237, 0.16358106938362343, 0.16417590242583022, 0.16417590242583022, 0.16437418010656563, 0.16437418010656563, 0.164572457787301, 0.164572457787301, 0.16536556851024348, 0.16496901314877238, 0.1647707354680367, 0.16496901314877238, 0.164572457787301, 0.1647707354680367, 0.16556384619097886, 0.164572457787301, 0.16496901314877238, 0.16516729082950807, 0.17309839805892913, 0.1778570623965821, 0.16833973372127642, 0.16655523459465643, 0.1667535122753921, 0.16655523459465643, 0.1661586792331856, 0.16576212387171455, 0.16576212387171455, 0.16556384619097886, 0.16596040155244995, 0.16536556851024348, 0.1647707354680367, 0.16496901314877238, 0.16437418010656563, 0.1647707354680367, 0.16516729082950807, 0.16556384619097886, 0.1661586792331856, 0.1669517899561275, 0.1669517899561275, 0.1671500676368629, 0.16754662299833398, 0.16734834531759857, 0.16754662299833398, 0.16814145604054076, 0.16833973372127642, 0.16853801140201183, 0.1691328444442183, 0.1689345667634829, 0.1691328444442183, 0.16952939980568937, 0.17012423284789616, 0.16952939980568937, 0.16952939980568937, 0.1689345667634829, 0.16873628908274751, 0.169331122124954, 0.1689345667634829, 0.169331122124954, 0.17012423284789616, 0.16992595516716075, 0.1719087319745159, 0.1715121766130448, 0.17171045429378018, 0.17210700965525128, 0.17210700965525128, 0.17210700965525128, 0.17250356501672237, 0.17290012037819374, 0.17349495342040022, 0.1736932311011356, 0.1740897864626067, 0.17468461950481345, 0.17508117486628455, 0.1758742855892267, 0.17567600790849103, 0.17666739631216857, 0.17627084095069806, 0.1760725632699621, 0.17627084095069806, 0.1758742855892267, 0.17627084095069806, 0.17627084095069806, 0.17666739631216857, 0.17686567399290426, 0.17706395167363964, 0.17726222935437505, 0.17765878471584612, 0.1784518954387886, 0.17884845080025968, 0.17924500616173045, 0.18003811688467292, 0.1802363945654083, 0.180434672246144, 0.18083122760761508, 0.18083122760761508, 0.1806329499268794, 0.18102950528835077, 0.18122778296908615, 0.18122778296908615, 0.18142606064982156, 0.18122778296908615, 0.18221917137276344, 0.18221917137276344, 0.18261572673423482, 0.18360711513791236, 0.18261572673423482, 0.18261572673423482, 0.18380539281864777, 0.18340883745717695, 0.18340883745717695, 0.18420194818011915, 0.18499505890306128, 0.1851933365837967, 0.18578816962600317, 0.18658128034894533, 0.18697783571041643, 0.18677955802968071, 0.19034855628292047, 0.19133994468659804, 0.1895554455599786, 0.1891588901985075, 0.18995200092144968, 0.1895554455599786, 0.18995200092144968, 0.20105555104263967, 0.200857273361904, 0.20184866176558156, 0.2030383278499945, 0.20422799393440805, 0.20482282697661452, 0.20541766001882128, 0.2050211046573499, 0.19471066525910236, 0.1923313330902759, 0.19133994468659804, 0.19292616613248237, 0.1923313330902759, 0.19193477772880452, 0.19252961077101155, 0.19272788845174696, 0.19292616613248237, 0.19332272149395344, 0.1937192768554245, 0.1943141098976313, 0.19352099917468912, 0.19292616613248237, 0.19292616613248237, 0.19490894293983776, 0.1937192768554245, 0.1937192768554245, 0.19471066525910236, 0.19471066525910236, 0.1964951643857218, 0.19590033134351562, 0.19590033134351562, 0.1962968867049864, 0.1962968867049864, 0.1960986090242513, 0.1966934420664575, 0.19550377598204483, 0.19550377598204483, 0.19471066525910236, 0.19332272149395344, 0.19292616613248237, 0.19272788845174696, 0.19272788845174696, 0.19272788845174696, 0.1937192768554245, 0.19252961077101155, 0.19133994468659804, 0.19133994468659804, 0.19114166700586294, 0.1915382223673337, 0.19133994468659804, 0.19133994468659804, 0.19114166700586294, 0.1915382223673337, 0.19094338932512753, 0.19114166700586294, 0.19133994468659804, 0.19054683396365615, 0.19034855628292047, 0.19114166700586294, 0.18995200092144968, 0.19034855628292047, 0.18995200092144968, 0.1895554455599786, 0.1893571678792429, 0.19074511164439184, 0.19015027860218509, 0.1895554455599786, 0.1891588901985075, 0.18896061251777183, 0.1891588901985075, 0.189753723240714, 0.189753723240714, 0.19114166700586294, 0.19054683396365615, 0.19015027860218509, 0.19133994468659804, 0.19094338932512753, 0.19094338932512753, 0.1915382223673337, 0.19292616613248237, 0.19272788845174696, 0.19272788845174696, 0.19332272149395344, 0.19391755453616022, 0.19471066525910236, 0.19490894293983776, 0.1957020536627802, 0.19550377598204483, 0.19530549830130883, 0.19550377598204483, 0.1960986090242513, 0.1957020536627802, 0.19550377598204483, 0.19530549830130883, 0.19550377598204483, 0.1957020536627802, 0.1962968867049864, 0.1966934420664575, 0.1966934420664575, 0.19708999742792888, 0.19728827510866426, 0.19827966351234183, 0.19788310815087073, 0.19808138583160642, 0.19986588495822616, 0.19907277423528427, 0.19907277423528427, 0.20581421538029238, 0.21255565652530017, 0.2030383278499945, 0.20125382872337477, 0.20145210640411018, 0.20165038408484587, 0.20224521712705262, 0.20165038408484587, 0.200857273361904, 0.20105555104263967, 0.200857273361904, 0.2006589956811686, 0.20165038408484587, 0.2004607180004329, 0.20105555104263967, 0.2004607180004329, 0.2004607180004329, 0.200857273361904, 0.20165038408484587, 0.20224521712705262, 0.20204693944631724, 0.2030383278499945, 0.20363316089220157, 0.20363316089220157, 0.20422799393440805, 0.20442627161514343, 0.2050211046573499, 0.20541766001882128, 0.20581421538029238, 0.20660732610323396, 0.20680560378396995, 0.20680560378396995, 0.20720215914544102, 0.2075987145069118, 0.20680560378396995, 0.20700388146470533, 0.2079952698683829, 0.20720215914544102, 0.20740043682617643, 0.20720215914544102, 0.20740043682617643, 0.20839182522985428, 0.2079952698683829, 0.20878838059132535, 0.2097797689950029, 0.2091849359527964, 0.2099780466757386, 0.21057287971794508, 0.21077115739868074, 0.21057287971794508, 0.21077115739868074, 0.21057287971794508, 0.21077115739868074, 0.21116771276015156, 0.21176254580235832, 0.21096943507941615, 0.21096943507941615, 0.21156426812162263, 0.21255565652530017, 0.21255565652530017, 0.21295221188677127, 0.21315048956750726, 0.21334876724824264, 0.21315048956750726, 0.21374532260971374, 0.2141418779711845, 0.2141418779711845, 0.21394360029044912, 0.21434015565192022, 0.2145384333326556, 0.21493498869412697, 0.21493498869412697, 0.21572809941706914, 0.21513326637486235, 0.21493498869412697, 0.21513326637486235, 0.21572809941706914, 0.21493498869412697, 0.21473671101339128, 0.21473671101339128, 0.2145384333326556, 0.2145384333326556, 0.21513326637486235, 0.21552982173633345, 0.21572809941706914, 0.2163229324592756, 0.21671948782074668, 0.21671948782074668, 0.21592637709780454, 0.2163229324592756, 0.21810743158589535, 0.2169177655014821, 0.21751259854368857, 0.218305709266631, 0.21850398694736642, 0.218305709266631, 0.21969365303177968, 0.21949537535104396, 0.22009020839325075, 0.22167642983913477, 0.22465059505016804, 0.22108159679692801, 0.22048676375472182, 0.21989193071251534, 0.221279874477664, 0.22068504143545722, 0.23119375851444046, 0.23079720315296937, 0.23059892547223398, 0.23218514691811803, 0.23337481300253154, 0.2353575898098867, 0.2345644790869448, 0.23159031387591156, 0.2236592066464902, 0.22227126288134155, 0.22207298520060587, 0.22266781824281234, 0.22286609592354834, 0.22187470751987048, 0.22207298520060587, 0.22286609592354834, 0.22266781824281234, 0.22266781824281234, 0.22266781824281234, 0.22266781824281234, 0.22266781824281234, 0.22246954056207696, 0.2232626512850194, 0.22266781824281234, 0.22286609592354834, 0.22246954056207696, 0.22207298520060587, 0.22246954056207696, 0.22187470751987048, 0.22187470751987048, 0.22266781824281234, 0.22207298520060587, 0.22246954056207696, 0.22306437360428372, 0.22246954056207696, 0.22246954056207696, 0.2254437057731102, 0.22306437360428372, 0.2232626512850194, 0.22266781824281234, 0.2236592066464902, 0.2234609289657548, 0.2236592066464902, 0.2236592066464902, 0.2240557620079613, 0.22306437360428372, 0.2234609289657548, 0.22385748432722588, 0.22385748432722588, 0.2236592066464902, 0.22385748432722588, 0.22425403968869667, 0.22385748432722588, 0.22445231736943266, 0.22524542809237452, 0.22484887273090373, 0.22504715041163914, 0.22524542809237452, 0.22564198345384562, 0.22683164953825885, 0.22683164953825885, 0.22722820489972964, 0.22762476026120101, 0.22841787098414318, 0.22861614866487856, 0.22940925938782103, 0.22881442634561397, 0.22881442634561397, 0.22940925938782103, 0.2296075370685564, 0.22980581474929182, 0.2304006477914986, 0.2304006477914986, 0.2304006477914986, 0.23198686923738263, 0.23099548083370508, 0.23159031387591156, 0.23079720315296937, 0.23059892547223398, 0.23079720315296937, 0.23119375851444046, 0.23099548083370508, 0.23139203619517615, 0.23178859155664694, 0.23198686923738263, 0.23218514691811803, 0.23317653532179589, 0.2325817022795894, 0.23198686923738263, 0.23198686923738263, 0.23139203619517615, 0.23198686923738263, 0.23099548083370508, 0.23059892547223398, 0.23079720315296937, 0.23059892547223398, 0.22980581474929182, 0.2302023701107629, 0.22980581474929182, 0.22940925938782103, 0.22980581474929182, 0.2296075370685564, 0.22901270402634966, 0.22901270402634966, 0.22881442634561397, 0.2296075370685564, 0.2296075370685564, 0.23396964604473802, 0.24090936487048242, 0.23337481300253154, 0.23139203619517615, 0.23099548083370508, 0.23119375851444046, 0.23099548083370508, 0.23059892547223398, 0.23099548083370508, 0.23119375851444046, 0.23139203619517615, 0.23159031387591156, 0.23178859155664694, 0.23218514691811803, 0.23119375851444046, 0.23119375851444046, 0.23139203619517615, 0.23178859155664694, 0.23178859155664694, 0.23198686923738263, 0.23198686923738263, 0.2325817022795894, 0.23317653532179589, 0.2327799799603248, 0.23297825764106048, 0.23337481300253154, 0.2345644790869448, 0.23496103444841587, 0.23496103444841587, 0.2353575898098867, 0.23615070053282883, 0.23555586749062235, 0.23595242285209345, 0.23654725589429992, 0.23654725589429992, 0.23654725589429992, 0.23753864429797805, 0.2373403666172421, 0.23753864429797805, 0.23793519965944915, 0.23912486574386238, 0.23971969878606886, 0.24051280950901105, 0.24090936487048242, 0.24130592023195319, 0.24190075327415966, 0.24229730863563076, 0.24289214167783724, 0.24289214167783724, 0.2436852524007794, 0.24447836312372184, 0.24428008544298618, 0.24428008544298618, 0.24408180776225077, 0.24447836312372184, 0.2436852524007794, 0.24328869703930833, 0.24309041935857292, 0.24289214167783724, 0.24309041935857292, 0.2438835300815151, 0.24289214167783724, 0.243486974720044, 0.24309041935857292, 0.24328869703930833, 0.243486974720044, 0.2436852524007794, 0.2436852524007794, 0.24428008544298618, 0.24487491848519266, 0.24487491848519266, 0.24527147384666373, 0.24606458456960617, 0.24546975152739942, 0.24546975152739942, 0.2458663068888705, 0.24546975152739942, 0.24467664080445725, 0.24408180776225077, 0.2438835300815151, 0.24328869703930833, 0.24309041935857292, 0.24209903095489538, 0.2415041979126889, 0.2411076425512178, 0.24090936487048242, 0.24170247559342428, 0.2407110871897467, 0.24051280950901105, 0.24090936487048242, 0.24051280950901105, 0.24170247559342428, 0.24130592023195319, 0.24090936487048242, 0.2415041979126889, 0.24190075327415966, 0.24269386399710186, 0.24289214167783724, 0.24309041935857292, 0.24289214167783724, 0.24309041935857292, 0.24765080601549022, 0.24309041935857292, 0.24289214167783724, 0.24249558631636645, 0.24209903095489538, 0.24269386399710186, 0.25201291499167244, 0.2506249712265235, 0.25121980426873, 0.25201291499167244, 0.25280602571461397, 0.2534008587568205, 0.25518535788344077, 0.25518535788344077, 0.25617674628711834, 0.25280602571461397, 0.25240947035314293, 0.2530043033953494, 0.25359913643755644, 0.254590524841234, 0.25141808194946536, 0.25141808194946536, 0.2534008587568205, 0.24249558631636645, 0.24031453182827534, 0.23912486574386238, 0.238728310382391, 0.23833175502091994, 0.23813347734018453, 0.23753864429797805, 0.23694381125577102, 0.23654725589429992, 0.23694381125577102, 0.2367455335750353, 0.2373403666172421, 0.2367455335750353, 0.23615070053282883, 0.23714208893650698, 0.23634897821356424, 0.23634897821356424, 0.23595242285209345, 0.23634897821356424, 0.23595242285209345, 0.2373403666172421, 0.23555586749062235, 0.23555586749062235, 0.23515931212915128, 0.2345644790869448, 0.2343662014062094, 0.23476275676768021, 0.2343662014062094, 0.23337481300253154, 0.23377136836400236, 0.2327799799603248, 0.2325817022795894, 0.23159031387591156, 0.23079720315296937, 0.22980581474929182, 0.22921098170708504, 0.22881442634561397, 0.2282195933034075, 0.22762476026120101, 0.22663337185752316, 0.2262368164960521, 0.22584026113458128, 0.22564198345384562, 0.22584026113458128, 0.22524542809237452, 0.22425403968869667, 0.22306437360428372, 0.22286609592354834, 0.22227126288134155, 0.2208833191161929, 0.22068504143545722, 0.21969365303177968, 0.2189005423088375, 0.21810743158589535, 0.21751259854368857, 0.21652121014001102, 0.21533154405559807, 0.21434015565192022, 0.21434015565192022, 
